vi "testi2.vi"() -> ()   [LabVIEW 2015]
uses:
  BERTTA.dll
panel:
  in  "mettler":dbl
  in  "lauda":dbl
  in  "heidolph":i32
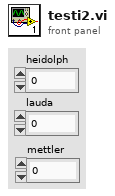
[diagram p1: front panel]
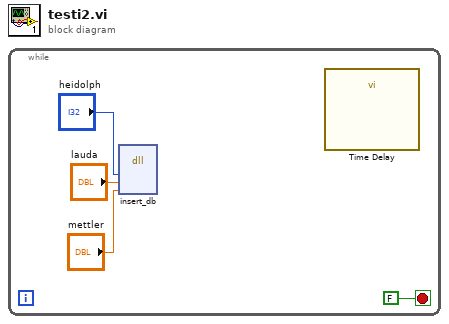
[diagram p0: block diagram]
diagram:
  n1 = while {
    stop <- FALSE stop-if-true
    n2 = dll-call lib="C:/Users/xlaraser/Documents/Visual Studio 2017/Projects/Bertta/BERTTA/Debug/BERTTA.dll" fn="insert_db"("heidolph"="heidolph", "lauda"="lauda", "mettler"="mettler") -> ()  [unwired: 7 in, 2 out]
    n3 = call "Time Delay"() -> ()  [unwired: 11 in, 1 out]
  }
